vi "Launch MainTop - Copy.vi"   [LabVIEW 2021]
uses:
  C:/Program Files (x86)/National Instruments/LabVIEW 2021/project/Create Actor from Template/_MCLB_Template/MCLB_Template.lvclass
  C:/Program Files (x86)/National Instruments/LabVIEW 2021/vi.lib/ActorFramework/Actor/Actor.lvclass
  <vilib>/ActorFramework/Actor/Actor.lvclass
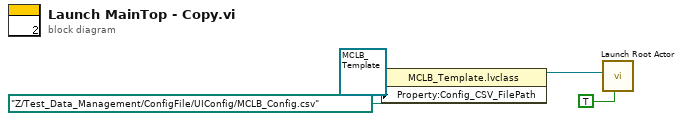
[diagram p0: block diagram]
diagram:
  n1 = property class="MCLB_Template.lvclass"(reference=refnum<class "MCLB_Template.lvclass"> refnum ("MCLB_Template.lvclass"), "Property:Config_CSV_FilePath"=path "Z:/Test_Data_Management/ConfigFile/UIConfig/MCLB_Config.csv" ("Config_CSV_FilePath")) -> (reference out=w3:refnum<class "MCLB_Template.lvclass">)  [unwired: 1 in, 1 out]
  n2 = call <vilib>:"Launch Root Actor.vi"("Open Actor Core front panel? (F)"=TRUE, "Actor"=w3) -> ()  [unwired: 8 in, 2 out]
